vi "Write Value.vi"(8 "error in (no error)":errorcluster, 9 "Value":variant, 10 "Key":i32, 11 "Integer Dictionary in":refnum<class "Integer Dictionary.lvclass">) -> (0 "error out":errorcluster, 2 "replaced?":bool, 3 "Integer Dictionary out":refnum<class "Integer Dictionary.lvclass">)   [LabVIEW 2013, in "Integer Dictionary.lvclass"]
uses:
  Integer Dictionary.lvclass
  Integer Dictionary.lvclass/Integer Dictionary.ctl
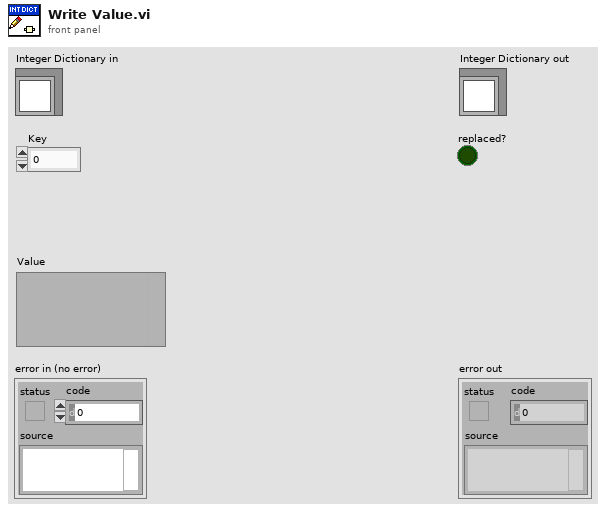
[diagram p1: front panel]
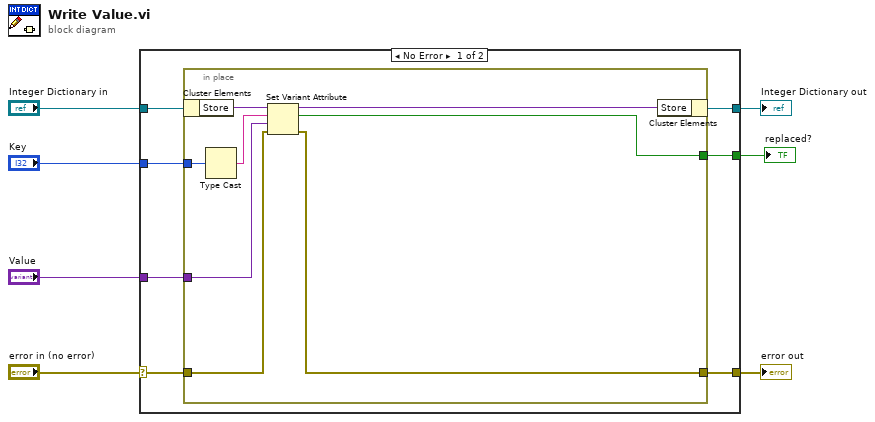
[diagram p0: block diagram]
diagram:
  n1 = case shown="No Error" "error in (no error)" {
    selector: "error in (no error)" -> [w12 w24]
    tunnel: [w11 w24] -> w6
    tunnel: [w13 w23] -> w4
    tunnel: "Integer Dictionary in" -> [w14 w23]
    tunnel: "Key" -> [w10 _]
    tunnel: "Value" -> [w9 _]
    tunnel: [w8 _] -> w1
    frame No Error {
      n2 = in-place {
        in-place-border: w12 -> [w20]
        in-place-border: [w19] -> w11
        in-place-border: w10 -> [w18]
        in-place-border: w9 -> [w16]
        in-place-border: [w15] -> w8
        n3 = in-place-cluster #1(w14) -> ("Store"=w22:variant)
        n4 = Type Cast(x=w18) -> (*(type *) &x=w17:string)  [unwired: 1 in]
        n5 = Set Variant Attribute(Variant=w22, name=w17, value=w16, error in=w20) -> (Variant out=w21:variant, replaced=w15:bool, error out=w19:errorcluster)
        n6 = in-place-cluster #1("Store"=w21) -> (w13:refnum<class "Integer Dictionary.lvclass">)
      }
    }
    frame Error {
    }
  }
  "error out" <- w6
  "Integer Dictionary out" <- w4
  "replaced?" <- w1
